vi "niRFUtil RFHS Util Get Errors.vi"() -> (4 "error cnt":u32, 6 "error codes":i32[](array[numeric]) format="%08x", 15 "error out":errorcluster)   [LabVIEW 2015, in "niRFUtil.lvlib"]
uses:
  niRFUtil.lvlib
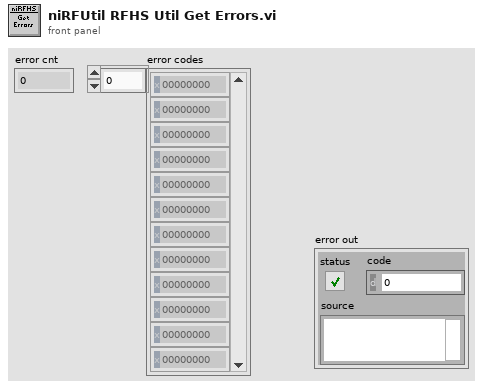
[diagram p1: front panel]
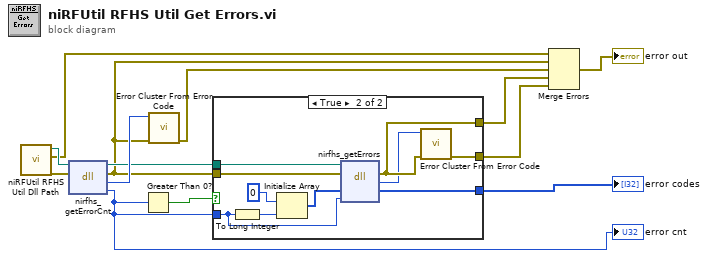
[diagram p0: block diagram]
diagram:
  n1 = call "niRFUtil RFHS Util Dll Path.vi"() -> ("error out"=w8:errorcluster, "Path"=w10:path)  [unwired: 7 in, 3 out]
  n2 = dll-call lib="M:/RfProtocols/RFmx/DLLs/niRFHS/trunk/2.0/dist/win32U/niRFHS_generic.*" fn="nirfhs_getErrorCnt"(path in=w10, error in=w8) -> (path out=w9:path, error out=w6:errorcluster, "return type"=w11:i32, "cnt"=w1:u32)  [unwired: 2 in]
  "error cnt" <- w1
  n3 = Greater Than 0?(x=w1) -> (x > 0?=w2:bool)
  n4 = call <vilib>:"Error Cluster From Error Code.vi"("error in (no error)"=w6, "error code (0)"=w11) -> ("error out"=w7:errorcluster)  [unwired: 7 in]
  n5 = case shown="True" w2 {
    tunnel: w9 -> [_ w21]
    tunnel: w1 -> [_ w18]
    tunnel: w6 -> [_ w17]
    tunnel: [_ w16] -> w5
    tunnel: [_ w15] -> w4
    tunnel: [_ w13] -> w3
    frame False {
    }
    frame True {
      n6 = To Long Integer(number=w18) -> (32bit integer=w20:i32)
      n7 = Initialize Array(0 ("element"), w20) -> (w19:i32[])
      n8 = dll-call lib="M:/RfProtocols/RFmx/DLLs/niRFHS/trunk/2.0/dist/win32U/niRFHS_generic.*" fn="nirfhs_getErrors"(path in=w21, error in=w17, "buf"=w19, "BufSize"=w18) -> (error out=w16:errorcluster, "return type"=w14:i32, "buf"=w13:i32[])  [unwired: 2 in, 1 out]
      n9 = call <vilib>:"Error Cluster From Error Code.vi"("error in (no error)"=w16, "error code (0)"=w14) -> ("error out"=w15:errorcluster)  [unwired: 7 in]
    }
  }
  "error codes" <- w3
  n10 = Merge Errors(w8, w6, w7, w5, w4) -> (→"error out":errorcluster)
